vi "Set Properties.vi"(8 "Error In":errorcluster, 10 "Properties":T1={"Font Name"="Segoe UI", "Size"=20.0, "Style"=enum."Regular", "Align"=1, "FG Color"=0, "BG Color"=16777215} {"Align" items=["TopLeft"=1, "TopCenter"=2, "TopRight"=4, "MiddleLeft"=16, "MiddleCenter"=32, "MiddleRight"=64, "BottomLeft"=256, "BottomCenter"=512, "BottomRight"=1024]}, 11 "Label In":refnum<k24>) -> (0 "Error Out":errorcluster, 3 "Label Out":refnum<k24>)   [LabVIEW 2020, in "Dot Net UI Controls.lvlib"]
uses:
  Dot Net UI Controls.lvlib
  System.Windows.Forms
  Label Properties.ctl
  Font Style.ctl
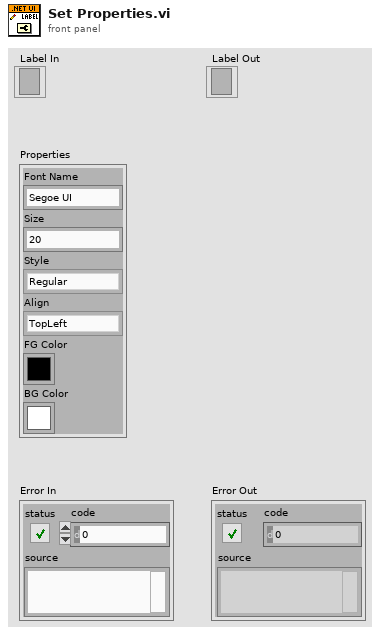
[diagram p1: front panel]
types:
  T1 = typedef "Dot Net UI Controls.lvlib/Label Properties.ctl" = cluster{"Font Name":string, "Size":sgl, "Style":T2, "Align":i32, "FG Color":u32, "BG Color":u32}
  T2 = typedef "Dot Net UI Controls.lvlib/Font Style.ctl" = enum16{"Regular", "Bold", "Italic", "Underline", "Strikeout"}
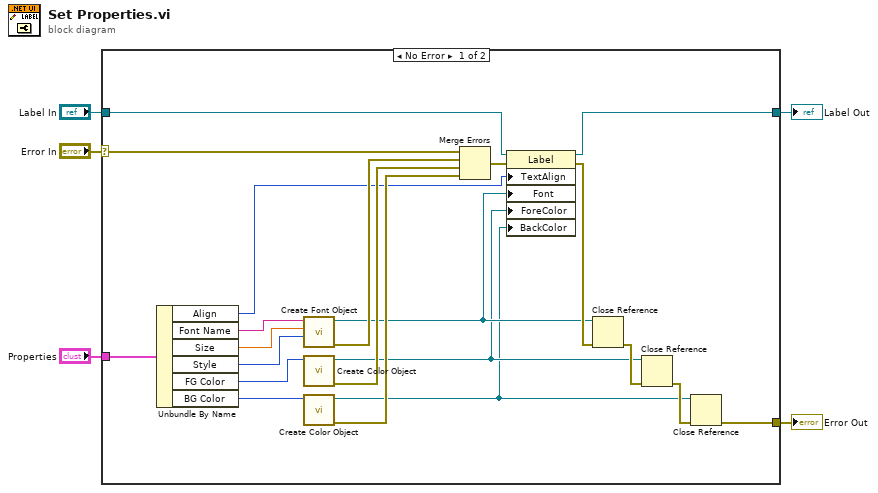
[diagram p0: block diagram]
diagram:
  n1 = case shown="No Error" "Error In" {
    selector: "Error In" -> [w6 w27]
    tunnel: [w22 w28] -> w5
    tunnel: "Label In" -> [w21 w28]
    tunnel: [w17 w27] -> w1
    tunnel: "Properties" -> [w13 _]
    frame No Error {
      n2 = Unbundle By Name(w13) -> ("Align"=w12:i32, "Font Name"=w11:string, "Size"=w10:sgl, "Style"=w9:T2, "FG Color"=w8:u32, "BG Color"=w7:u32)
      n3 = call "Create Font Object.vi"("Style"=w9, "Size"=w10, "Name"=w11) -> ("Error Out"=w25:errorcluster, "Font Object"=w20:refnum<k24>)  [unwired: 7 in]
      n4 = call "Create Color Object.vi"("Color (black)"=w8) -> ("Error Out"=w24:errorcluster, "Color Object"=w16:refnum<k24>)  [unwired: 9 in]
      n5 = call "Create Color Object.vi"("Color (black)"=w7) -> ("Error Out"=w23:errorcluster, "Color Object"=w15:refnum<k24>)  [unwired: 9 in]
      n6 = Merge Errors(w6, w25, w24, w23) -> (w14:errorcluster)
      n7 = property class="Label"(reference=w21, error in=w14, "TextAlign"=w12, "Font"=w20, "ForeColor"=w16, "BackColor"=w15) -> (reference out=w22:refnum<k24>, error out=w26:errorcluster)
      n8 = Close Reference(reference=w20, error in (no error)=w26) -> (error out=w18:errorcluster)
      n9 = Close Reference(reference=w16, error in (no error)=w18) -> (error out=w19:errorcluster)
      n10 = Close Reference(reference=w15, error in (no error)=w19) -> (error out=w17:errorcluster)
    }
    frame Error {
    }
  }
  "Label Out" <- w5
  "Error Out" <- w1
